vi "AccelerometerTest.vi"() -> ()   [LabVIEW 2016]
uses:
  Telemetry/TelemetryFields.ctl
  <vilib>/rvi/Emulation/niFpgaGetClockAttributes.vi
  <vilib>/rvi/Emulation/niFpgaSctlEmulationGetInTimedLoop.vi
  <vilib>/rvi/Emulation/niFpgaEmulationReportErrorSimple.vi
  <vilib>/rvi/Emulation/niFpgaEmulationIsFPGAContextNoSignature.vi
  <vilib>/rvi/errors/niFpgaSetErrorForExecOnDevCompSimple.vi
  <vilib>/rvi/eio/common/nirviEmuReportErrorAndStop.vi
  <vilib>/rvi/DataTransferAndStorage/Container/Common/niFpgaContainerGetUniqueNameForEmu.vi
  <vilib>/rvi/FIFO/Fifo_Resource/nirvififoEmulationSetSize.vi
  <vilib>/rvi/FIFO/Fifo_Resource/nirviFifoEmulationQueueMgr.vi
  <instcachedir>/0/nirviFifoEmulationQueueMgr_E5CAEC123FF24DC58D834DCA3CDAA9B5.lvgen/nirviFifoEmulationQueueMgr_E5CAEC123FF24DC58D834DCA3CDAA9B5_004.vi
  <vilib>/rvi/FIFO/Fifo_Resource/nirvififoEmulationDetermineInputValidOut.vi
  <vilib>/rvi/FIFO/Fifo_Resource/nirvififoEmulationCreateLock.vi
  <vilib>/rvi/Emulation/niFpgaProcessEmulError.vi
  <vilib>/rvi/FIFO/Fifo_Resource/nirvififoEmulationObtainLock.vi
  <vilib>/rvi/FIFO/Fifo_Resource/nirvififoEmulationReleaseLock.vi
  <vilib>/rvi/occurrence/nirviWaitOnOccurrenceBase.vi
  <vilib>/rvi/errors/nirviReportUnexpectedCaseInternalError.vi
  <vilib>/rvi/errors/nirviReportUnexpectedCaseInternalError (U32).vi
  <vilib>/Utility/error.llb/Clear Errors.vi
  <vilib>/rvi/Emulation/niFpgaCriticalErrorInLSC.vi
  <instcachedir>/0/nirviFifoEmulationQueueMgr_E5CAEC123FF24DC58D834DCA3CDAA9B5.lvgen/nirviFifoEmulationQueueMgr_E5CAEC123FF24DC58D834DCA3CDAA9B5_038.vi
  <instcachedir>/0/nirviFifoEmulationQueueMgr_E5CAEC123FF24DC58D834DCA3CDAA9B5.lvgen/nirviFifoEmulationQueueMgr_E5CAEC123FF24DC58D834DCA3CDAA9B5_039.vi
  <instcachedir>/0/nirviFifoEmulationQueueMgr_E5CAEC123FF24DC58D834DCA3CDAA9B5.lvgen/nirviFifoEmulationQueueMgr_E5CAEC123FF24DC58D834DCA3CDAA9B5_029.vi
  <instcachedir>/0/nirviFifoEmulationQueueMgr_E5CAEC123FF24DC58D834DCA3CDAA9B5.lvgen/nirviFifoEmulationQueueMgr_E5CAEC123FF24DC58D834DCA3CDAA9B5_028.vi
  <instcachedir>/0/nirviFifoEmulationQueueMgr_E5CAEC123FF24DC58D834DCA3CDAA9B5.lvgen/nirviFifoEmulationQueueMgr_E5CAEC123FF24DC58D834DCA3CDAA9B5_033.vi
  <instcachedir>/0/nirviFifoEmulationQueueMgr_E5CAEC123FF24DC58D834DCA3CDAA9B5.lvgen/nirviFifoEmulationQueueMgr_E5CAEC123FF24DC58D834DCA3CDAA9B5_035.vi
  <instcachedir>/0/nirviFifoEmulationQueueMgr_E5CAEC123FF24DC58D834DCA3CDAA9B5.lvgen/nirviFifoEmulationQueueMgr_E5CAEC123FF24DC58D834DCA3CDAA9B5_043.vi
  <instcachedir>/0/nirviFifoEmulationQueueMgr_E5CAEC123FF24DC58D834DCA3CDAA9B5.lvgen/nirviFifoEmulationQueueMgr_E5CAEC123FF24DC58D834DCA3CDAA9B5_041.vi
  <instcachedir>/0/nirviFifoEmulationQueueMgr_E5CAEC123FF24DC58D834DCA3CDAA9B5.lvgen/nirviFifoEmulationQueueMgr_E5CAEC123FF24DC58D834DCA3CDAA9B5_042.vi
  <instcachedir>/0/nirviFifoEmulationQueueMgr_E5CAEC123FF24DC58D834DCA3CDAA9B5.lvgen/nirviFifoEmulationQueueMgr_E5CAEC123FF24DC58D834DCA3CDAA9B5_040.vi
  <vilib>/rvi/DataTransferAndStorage/Container/XNode/niFpgaContainer.xnode
  <vilib>/rvi/FIFO/Fifo_Resource/nirvififoEmulationWrite.vi
  <vilib>/rvi/FIFO/Fifo_Resource/nirvififoEmulationRead.vi
panel:
  out "AngularAccelerationZ":sgl format="%#.6f"
  out "AngularAccelerationY":sgl format="%#.6f"
  out "AngularAccelerationX":sgl format="%#.6f"
  out "AccelerometerEng8":sgl format="%#.6f"
  out "AccelerometerEng7":sgl format="%#.6f"
  out "AccelerometerEng6":sgl format="%#.6f"
  out "AccelerometerEng5":sgl format="%#.6f"
  out "AccelerometerEng4":sgl format="%#.6f"
  out "AccelerometerEng3":sgl format="%#.6f"
  out "AccelerometerEng2":sgl format="%#.6f"
  out "AccelerometerEng1":sgl format="%#.6f"
  out "AccelerometerTimestamp":u64
  out "AccelerometerRaw1":sgl format="%#.6f"
  out "AccelerometerRaw2":sgl format="%#.6f"
  out "AccelerometerRaw3":sgl format="%#.6f"
  out "AccelerometerRaw4":sgl format="%#.6f"
  out "AccelerometerRaw5":sgl format="%#.6f"
  out "AccelerometerRaw6":sgl format="%#.6f"
  out "AccelerometerRaw7":sgl format="%#.6f"
  out "AccelerometerRaw8":sgl format="%#.6f"
  out "AccelerometerSampleCount":u64
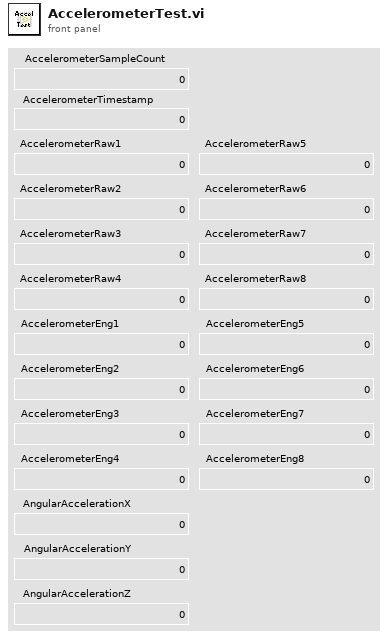
[diagram p1: front panel]
types:
  T1 = cluster{"Timestamp":u64, "TxBytes":u64, "RxBytes":u64, "TxFrames":u64, "RxFrames":u64, "BIT0":u8, "BIT1":u8, "BIT2":u8, "BIT3":u8, "BIT4":u8, "BIT5":u8}
  T2 = cluster{"Timestamp":u64, "TxBytes":u64, "RxBytes":u64, "TxFrames":u64, "RxFrames":u64, "GyroX":u32, "GyroY":u32, "GyroZ":u32, "Status":u8, "SequenceNumber":u8, "Temperature":i16}
  T3 = cluster{"Timestamp":u64, "TxBytes":u64, "RxBytes":u64, "TxFrames":u64, "RxFrames":u64, "BIT0":u8, "BIT1":u8, "BIT2":u8, "BIT3":u8, "BIT4":u8, "BIT5":u8, "BIT6":u8, "BIT7":u8}
  T4 = cluster{"Timestamp":u64, "TxBytes":u64, "RxBytes":u64, "TxFrames":u64, "RxFrames":u64, "ErrorCode":enum8{"None", "ResponseHeaderError", "ResponseCRCError", "ResponseTimeoutError", "ResponseChecksumError"}}
  T5 = cluster{"Timestamp":u64, "TxBytes":u64, "RxBytes":u64, "TxFrames":u64, "RxFrames":u64, "RawAngle":i32, "ZenithAngle":sgl}
  T6 = cluster{"Timestamp":u64, "TxBytes":u64, "RxBytes":u64, "TxFrames":u64, "RxFrames":u64, "ErrorCode":enum8{"None", "ResponseAddressError", "ResponseFunctionCodeError", "ResponseByteCountError", "ResponseCRCError", "ResponseUnknownError", "ResponseTimeoutError", "SensorReportsIllegalFunction", "SensorReportsIllegalDataAddress"}}
  T7 = cluster{"Timestamp":u64, "TxBytes":u64, "RxBytes":u64, "TxFrames":u64, "RxFrames":u64, "Sensor1Raw":i32, "Sensor2Raw":i32, "Sensor3Raw":i32, "Sensor4Raw":i32, "Sensor5Raw":i32, "Sensor6Raw":i32, "Sensor7Raw":i32, "Sensor8Raw":i32, "Sensor1Eng":sgl, "Sensor2Eng":sgl, "Sensor3Eng":sgl, "Sensor4Eng":sgl, "Sensor5Eng":sgl, "Sensor6Eng":sgl, "Sensor7Eng":sgl, "Sensor8Eng":sgl, "PositionX":sgl, "PositionY":sgl, "PositionZ":sgl, "RotationX":sgl, "RotationY":sgl, "RotationZ":sgl}
  T8 = cluster{"Timestamp":u64, "TxBytes":u64, "RxBytes":u64, "TxFrames":u64, "RxFrames":u64, "ErrorCode":enum16{"None", "ResponseUnknownError", "ResponseInvalidError", "ResponseTimeoutError", "SensorIndicatesInvalidCommandError", "SensorIndicatesCommunicationTimeoutError", "SensorIndicatesDataLengthError", "SensorIndicatesNumberOfParametersError", "SensorIndicatesParameterError", "SensorIndicatesCommunicationError", "SensorIndicatesIDNumberError", "SensorIndicatesExpansionLineError", "SensorIndicatesWriteControlError"}}
  T9 = typedef "TelemetryFields.ctl" = enum16{"None", "InclinometerTxBytes", "InclinometerRxBytes", "InclinometerTxFrames", "InclinometerRxFrames", "InclinometerErrorTimestamp", "InclinometerErrorCode", "InclinometerSampleTimestamp", "InclinometerRawAngle", "InclinometerZenithAngle", "DisplacementTxBytes", "DisplacementRxBytes", "DisplacementTxFrames", "DisplacementRxFrames", "DisplacementErrorTimestamp", "DisplacementErrorCode", "DisplacementSampleTimestamp", "DisplacementRaw1", "DisplacementRaw2", "DisplacementRaw3", "DisplacementRaw4", "DisplacementRaw5", "DisplacementRaw6", "DisplacementRaw7", "DisplacementRaw8", "DisplacementEng1", "DisplacementEng2", "DisplacementEng3", "DisplacementEng4", "DisplacementEng5", "DisplacementEng6", "DisplacementEng7", "DisplacementEng8", "DisplacementPositionX", "DisplacementPositionY", "DisplacementPositionZ", "DisplacementRotationX", "DisplacementRotationY", "DisplacementRotationZ", "AccelerometerSampleCount", "AccelerometerSampleTimestamp", "AccelerometerRaw1", "AccelerometerRaw2", "AccelerometerRaw3", "AccelerometerRaw4", "AccelerometerRaw5", "AccelerometerRaw6", "AccelerometerRaw7", "AccelerometerRaw8", "AccelerometerEng1", "AccelerometerEng2", "AccelerometerEng3", "AccelerometerEng4", "AccelerometerEng5", "AccelerometerEng6", "AccelerometerEng7", "AccelerometerEng8", "AngularAccelerationX", "AngularAccelerationY", "AngularAccelerationZ", "GyroTxBytes", "GyroRxBytes", "GyroTxFrames", "GyroRxFrames", "GyroErrorTimestamp", "GyroErrorCode", "GyroSampleTimestamp", "AngularVelocityX", "AngularVelocityY", "AngularVelocityZ", "GyroStatus", "GyroSequenceNumber", "GyroTemperature", "GyroBITTimestamp", "GyroBIT0", "GyroBIT1", "GyroBIT2", "GyroBIT3", "GyroBIT4", "GyroBIT5", "GyroBIT6", "GyroBIT7"}
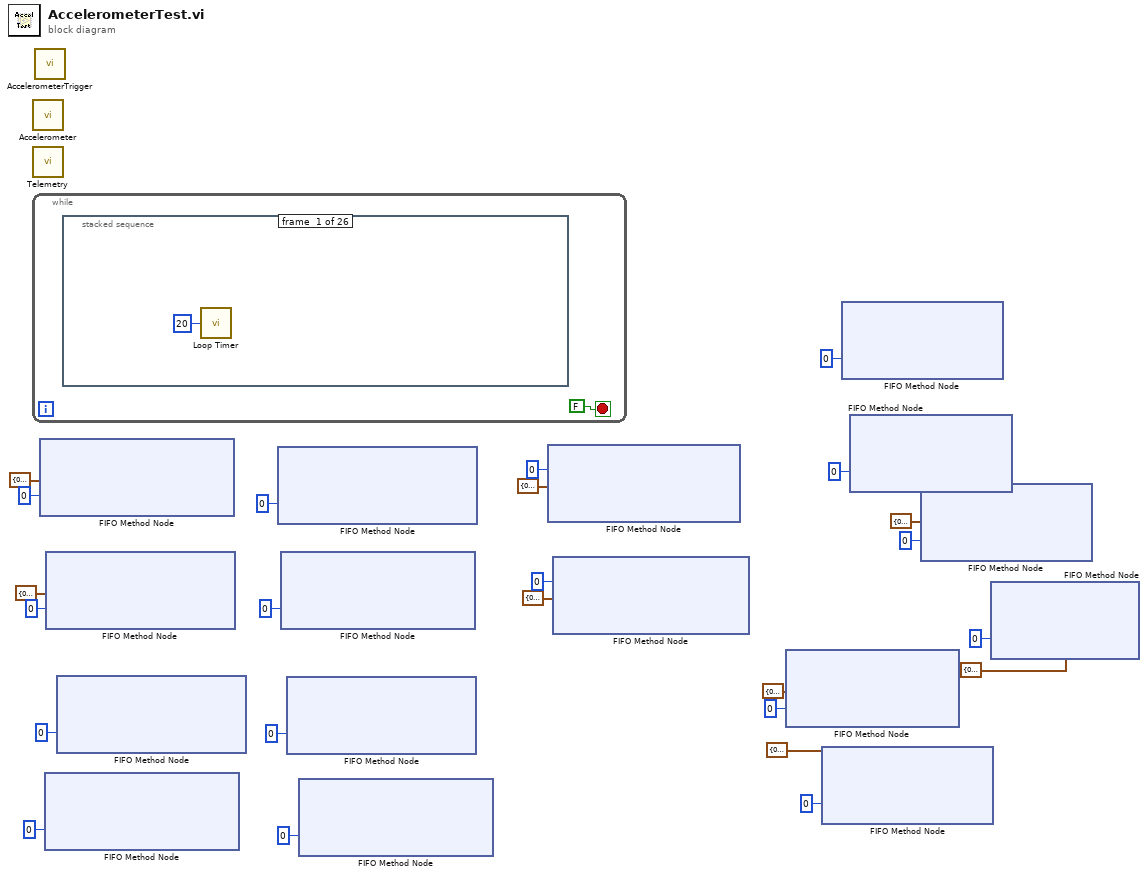
[diagram p0: block diagram]
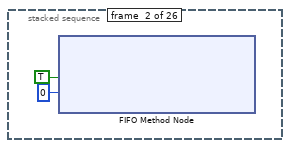
[diagram p2: hidden frame]
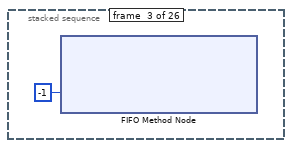
[diagram p3: hidden frame]
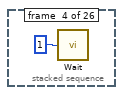
[diagram p4: hidden frame]
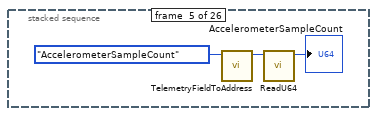
[diagram p5: hidden frame]
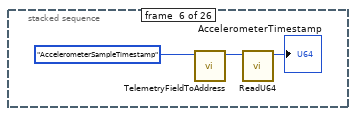
[diagram p6: hidden frame]
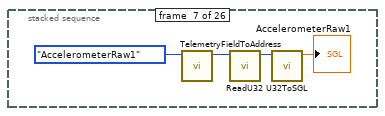
[diagram p7: hidden frame]
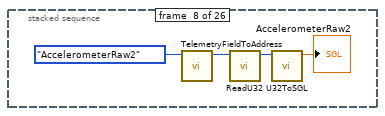
[diagram p8: hidden frame]
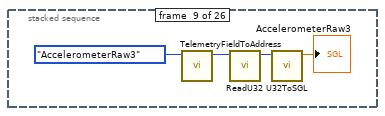
[diagram p9: hidden frame]
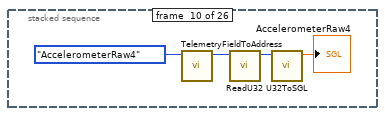
[diagram p10: hidden frame]
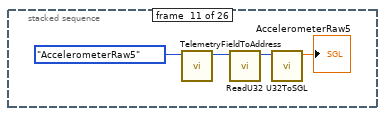
[diagram p11: hidden frame]
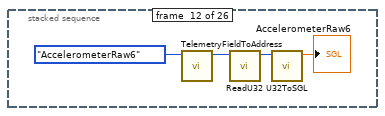
[diagram p12: hidden frame]
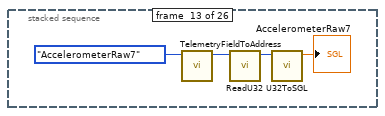
[diagram p13: hidden frame]
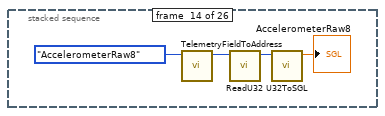
[diagram p14: hidden frame]
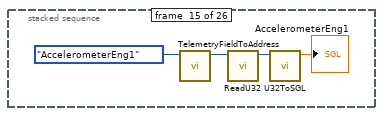
[diagram p15: hidden frame]
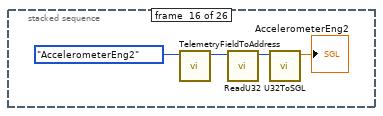
[diagram p16: hidden frame]
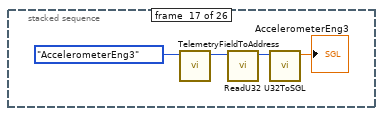
[diagram p17: hidden frame]
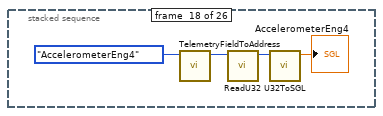
[diagram p18: hidden frame]
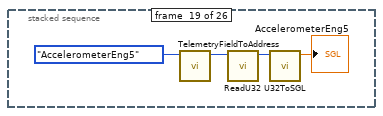
[diagram p19: hidden frame]
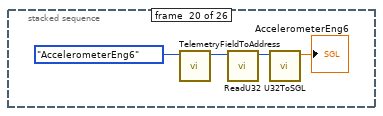
[diagram p20: hidden frame]
diagram:
  n1 = call "Accelerometer.vi"() -> ()  [unwired: 12 in]
  n2 = call "Telemetry.vi"() -> ()  [unwired: 12 in]
  n3 = while {
    stop <- FALSE stop-if-true
    n4 = stacked-sequence {
      frame #0 {
        n5 = call "Loop Timer"("Count(mSec)"=u8 20) -> ()  [unwired: 1 out]
      }
      frame #1 {
        n6 = xnode ("FIFO Method Node")("Element"=TRUE, "Timeout"=0) -> ()  [unwired: 1 in, 2 out]
      }
      frame #2 {
        n7 = xnode ("FIFO Method Node")("Timeout"=-1) -> ()  [unwired: 1 in, 3 out]
      }
      frame #3 {
        n8 = call "Wait"("Count(uSec)"=u8 1 ("Count(mSec)")) -> ()  [unwired: 1 out]
      }
      frame #4 {
        n9 = call "TelemetryFieldToAddress.vi"("TelemetryFields"=TelemetryFields."AccelerometerSampleCount") -> ("Address"=w32:u32)  [unwired: 10 in]
        n10 = call "ReadU64.vi"("Address"=w32) -> ("Data"=→"AccelerometerSampleCount":u64)  [unwired: 10 in]
      }
      frame #5 {
        n11 = call "TelemetryFieldToAddress.vi"("TelemetryFields"=TelemetryFields."AccelerometerSampleTimestamp") -> ("Address"=w36:u32)  [unwired: 10 in]
        n12 = call "ReadU64.vi"("Address"=w36) -> ("Data"=→"AccelerometerTimestamp":u64)  [unwired: 10 in]
      }
      frame #6 {
        n13 = call "TelemetryFieldToAddress.vi"("TelemetryFields"=TelemetryFields."AccelerometerRaw1") -> ("Address"=w40:u32)  [unwired: 10 in]
        n14 = call "ReadU32.vi"("Address"=w40) -> ("Data"=w39:u32)  [unwired: 10 in]
        n15 = call "U32ToSGL.vi"("U32"=w39) -> ("SGL"=→"AccelerometerRaw1":sgl)  [unwired: 10 in]
      }
      frame #7 {
        n16 = call "TelemetryFieldToAddress.vi"("TelemetryFields"=TelemetryFields."AccelerometerRaw2") -> ("Address"=w44:u32)  [unwired: 10 in]
        n17 = call "ReadU32.vi"("Address"=w44) -> ("Data"=w43:u32)  [unwired: 10 in]
        n18 = call "U32ToSGL.vi"("U32"=w43) -> ("SGL"=→"AccelerometerRaw2":sgl)  [unwired: 10 in]
      }
      frame #8 {
        n19 = call "TelemetryFieldToAddress.vi"("TelemetryFields"=TelemetryFields."AccelerometerRaw3") -> ("Address"=w48:u32)  [unwired: 10 in]
        n20 = call "ReadU32.vi"("Address"=w48) -> ("Data"=w47:u32)  [unwired: 10 in]
        n21 = call "U32ToSGL.vi"("U32"=w47) -> ("SGL"=→"AccelerometerRaw3":sgl)  [unwired: 10 in]
      }
      frame #9 {
        n22 = call "TelemetryFieldToAddress.vi"("TelemetryFields"=TelemetryFields."AccelerometerRaw4") -> ("Address"=w52:u32)  [unwired: 10 in]
        n23 = call "ReadU32.vi"("Address"=w52) -> ("Data"=w51:u32)  [unwired: 10 in]
        n24 = call "U32ToSGL.vi"("U32"=w51) -> ("SGL"=→"AccelerometerRaw4":sgl)  [unwired: 10 in]
      }
      frame #10 {
        n25 = call "TelemetryFieldToAddress.vi"("TelemetryFields"=TelemetryFields."AccelerometerRaw5") -> ("Address"=w56:u32)  [unwired: 10 in]
        n26 = call "ReadU32.vi"("Address"=w56) -> ("Data"=w55:u32)  [unwired: 10 in]
        n27 = call "U32ToSGL.vi"("U32"=w55) -> ("SGL"=→"AccelerometerRaw5":sgl)  [unwired: 10 in]
      }
      frame #11 {
        n28 = call "TelemetryFieldToAddress.vi"("TelemetryFields"=TelemetryFields."AccelerometerRaw6") -> ("Address"=w60:u32)  [unwired: 10 in]
        n29 = call "ReadU32.vi"("Address"=w60) -> ("Data"=w59:u32)  [unwired: 10 in]
        n30 = call "U32ToSGL.vi"("U32"=w59) -> ("SGL"=→"AccelerometerRaw6":sgl)  [unwired: 10 in]
      }
      frame #12 {
        n31 = call "TelemetryFieldToAddress.vi"("TelemetryFields"=TelemetryFields."AccelerometerRaw7") -> ("Address"=w64:u32)  [unwired: 10 in]
        n32 = call "ReadU32.vi"("Address"=w64) -> ("Data"=w63:u32)  [unwired: 10 in]
        n33 = call "U32ToSGL.vi"("U32"=w63) -> ("SGL"=→"AccelerometerRaw7":sgl)  [unwired: 10 in]
      }
      frame #13 {
        n34 = call "TelemetryFieldToAddress.vi"("TelemetryFields"=TelemetryFields."AccelerometerRaw8") -> ("Address"=w68:u32)  [unwired: 10 in]
        n35 = call "ReadU32.vi"("Address"=w68) -> ("Data"=w67:u32)  [unwired: 10 in]
        n36 = call "U32ToSGL.vi"("U32"=w67) -> ("SGL"=→"AccelerometerRaw8":sgl)  [unwired: 10 in]
      }
      frame #14 {
        n37 = call "TelemetryFieldToAddress.vi"("TelemetryFields"=TelemetryFields."AccelerometerEng1") -> ("Address"=w72:u32)  [unwired: 10 in]
        n38 = call "ReadU32.vi"("Address"=w72) -> ("Data"=w71:u32)  [unwired: 10 in]
        n39 = call "U32ToSGL.vi"("U32"=w71) -> ("SGL"=→"AccelerometerEng1":sgl)  [unwired: 10 in]
      }
      frame #15 {
        n40 = call "TelemetryFieldToAddress.vi"("TelemetryFields"=TelemetryFields."AccelerometerEng2") -> ("Address"=w76:u32)  [unwired: 10 in]
        n41 = call "ReadU32.vi"("Address"=w76) -> ("Data"=w75:u32)  [unwired: 10 in]
        n42 = call "U32ToSGL.vi"("U32"=w75) -> ("SGL"=→"AccelerometerEng2":sgl)  [unwired: 10 in]
      }
      frame #16 {
        n43 = call "TelemetryFieldToAddress.vi"("TelemetryFields"=TelemetryFields."AccelerometerEng3") -> ("Address"=w80:u32)  [unwired: 10 in]
        n44 = call "ReadU32.vi"("Address"=w80) -> ("Data"=w79:u32)  [unwired: 10 in]
        n45 = call "U32ToSGL.vi"("U32"=w79) -> ("SGL"=→"AccelerometerEng3":sgl)  [unwired: 10 in]
      }
      frame #17 {
        n46 = call "TelemetryFieldToAddress.vi"("TelemetryFields"=TelemetryFields."AccelerometerEng4") -> ("Address"=w84:u32)  [unwired: 10 in]
        n47 = call "ReadU32.vi"("Address"=w84) -> ("Data"=w83:u32)  [unwired: 10 in]
        n48 = call "U32ToSGL.vi"("U32"=w83) -> ("SGL"=→"AccelerometerEng4":sgl)  [unwired: 10 in]
      }
      frame #18 {
        n49 = call "TelemetryFieldToAddress.vi"("TelemetryFields"=TelemetryFields."AccelerometerEng5") -> ("Address"=w88:u32)  [unwired: 10 in]
        n50 = call "ReadU32.vi"("Address"=w88) -> ("Data"=w87:u32)  [unwired: 10 in]
        n51 = call "U32ToSGL.vi"("U32"=w87) -> ("SGL"=→"AccelerometerEng5":sgl)  [unwired: 10 in]
      }
      frame #19 {
        n52 = call "TelemetryFieldToAddress.vi"("TelemetryFields"=TelemetryFields."AccelerometerEng6") -> ("Address"=w92:u32)  [unwired: 10 in]
        n53 = call "ReadU32.vi"("Address"=w92) -> ("Data"=w91:u32)  [unwired: 10 in]
        n54 = call "U32ToSGL.vi"("U32"=w91) -> ("SGL"=→"AccelerometerEng6":sgl)  [unwired: 10 in]
      }
      frame #20 {
        n55 = call "TelemetryFieldToAddress.vi"("TelemetryFields"=TelemetryFields."AccelerometerEng7") -> ("Address"=w96:u32)  [unwired: 10 in]
        n56 = call "ReadU32.vi"("Address"=w96) -> ("Data"=w95:u32)  [unwired: 10 in]
        n57 = call "U32ToSGL.vi"("U32"=w95) -> ("SGL"=→"AccelerometerEng7":sgl)  [unwired: 10 in]
      }
      frame #21 {
        n58 = call "TelemetryFieldToAddress.vi"("TelemetryFields"=TelemetryFields."AccelerometerEng8") -> ("Address"=w100:u32)  [unwired: 10 in]
        n59 = call "ReadU32.vi"("Address"=w100) -> ("Data"=w99:u32)  [unwired: 10 in]
        n60 = call "U32ToSGL.vi"("U32"=w99) -> ("SGL"=→"AccelerometerEng8":sgl)  [unwired: 10 in]
      }
      frame #22 {
        n61 = call "TelemetryFieldToAddress.vi"("TelemetryFields"=TelemetryFields."AngularAccelerationX") -> ("Address"=w104:u32)  [unwired: 10 in]
        n62 = call "ReadU32.vi"("Address"=w104) -> ("Data"=w103:u32)  [unwired: 10 in]
        n63 = call "U32ToSGL.vi"("U32"=w103) -> ("SGL"=→"AngularAccelerationX":sgl)  [unwired: 10 in]
      }
      frame #23 {
        n64 = call "TelemetryFieldToAddress.vi"("TelemetryFields"=TelemetryFields."AngularAccelerationY") -> ("Address"=w108:u32)  [unwired: 10 in]
        n65 = call "ReadU32.vi"("Address"=w108) -> ("Data"=w107:u32)  [unwired: 10 in]
        n66 = call "U32ToSGL.vi"("U32"=w107) -> ("SGL"=→"AngularAccelerationY":sgl)  [unwired: 10 in]
      }
      frame #24 {
        n67 = call "TelemetryFieldToAddress.vi"("TelemetryFields"=TelemetryFields."AngularAccelerationZ") -> ("Address"=w112:u32)  [unwired: 10 in]
        n68 = call "ReadU32.vi"("Address"=w112) -> ("Data"=w111:u32)  [unwired: 10 in]
        n69 = call "U32ToSGL.vi"("U32"=w111) -> ("SGL"=→"AngularAccelerationZ":sgl)  [unwired: 10 in]
      }
      frame #25 {
        n70 = xnode ("FIFO Method Node")("Element"=TRUE, "Timeout"=0) -> ()  [unwired: 1 in, 2 out]
      }
    }
  }
  n71 = call "AccelerometerTrigger.vi"() -> ()  [unwired: 12 in]
  n72 = xnode ("FIFO Method Node")("Element"=T8 {"Timestamp"=0, "TxBytes"=0, "RxBytes"=0, "TxFrames"=0, "RxFrames"=0, "ErrorCode"=enum."None"}, "Timeout"=0) -> ()  [unwired: 1 in, 2 out]
  n73 = xnode ("FIFO Method Node")("Timeout"=0) -> ()  [unwired: 1 in, 3 out]
  n74 = xnode ("FIFO Method Node")("Element"=T6 {"Timestamp"=0, "TxBytes"=0, "RxBytes"=0, "TxFrames"=0, "RxFrames"=0, "ErrorCode"=enum."None"}, "Timeout"=0) -> ()  [unwired: 1 in, 2 out]
  n75 = xnode ("FIFO Method Node")("Timeout"=0) -> ()  [unwired: 1 in, 3 out]
  n76 = xnode ("FIFO Method Node")("Timeout"=0) -> ()  [unwired: 1 in, 3 out]
  n77 = xnode ("FIFO Method Node")("Timeout"=0) -> ()  [unwired: 1 in, 3 out]
  n78 = xnode ("FIFO Method Node")("Timeout"=0) -> ()  [unwired: 1 in, 3 out]
  n79 = xnode ("FIFO Method Node")("Timeout"=0) -> ()  [unwired: 1 in, 3 out]
  n80 = xnode ("FIFO Method Node")("Element"=T7 {"Timestamp"=0, "TxBytes"=0, "RxBytes"=0, "TxFrames"=0, "RxFrames"=0, "Sensor1Raw"=0, "Sensor2Raw"=0, "Sensor3Raw"=0, "Sensor4Raw"=0, "Sensor5Raw"=0, "Sensor6Raw"=0, "Sensor7Raw"=0, "Sensor8Raw"=0, "Sensor1Eng"=0.0, "Sensor2Eng"=0.0, "Sensor3Eng"=0.0, "Sensor4Eng"=0.0, "Sensor5Eng"=0.0, "Sensor6Eng"=0.0, "Sensor7Eng"=0.0, "Sensor8Eng"=0.0, "PositionX"=0.0, "PositionY"=0.0, "PositionZ"=0.0, "RotationX"=0.0, "RotationY"=0.0, "RotationZ"=0.0}, "Timeout"=0) -> ()  [unwired: 1 in, 2 out]
  n81 = xnode ("FIFO Method Node")("Element"=T5 {"Timestamp"=0, "TxBytes"=0, "RxBytes"=0, "TxFrames"=0, "RxFrames"=0, "RawAngle"=0, "ZenithAngle"=0.0}, "Timeout"=0) -> ()  [unwired: 1 in, 2 out]
  n82 = xnode ("FIFO Method Node")("Element"=T4 {"Timestamp"=0, "TxBytes"=0, "RxBytes"=0, "TxFrames"=0, "RxFrames"=0, "ErrorCode"=enum."None"}, "Timeout"=0) -> ()  [unwired: 1 in, 2 out]
  n83 = xnode ("FIFO Method Node")("Element"=T1 {"Timestamp"=0, "TxBytes"=0, "RxBytes"=0, "TxFrames"=0, "RxFrames"=0, "BIT0"=0, "BIT1"=0, "BIT2"=0, "BIT3"=0, "BIT4"=0, "BIT5"=0}, "Timeout"=0) -> ()  [unwired: 1 in, 2 out]
  n84 = xnode ("FIFO Method Node")("Timeout"=0) -> ()  [unwired: 1 in, 3 out]
  n85 = xnode ("FIFO Method Node")("Timeout"=0) -> ()  [unwired: 1 in, 3 out]
  n86 = xnode ("FIFO Method Node")("Element"=T3 {"Timestamp"=0, "TxBytes"=0, "RxBytes"=0, "TxFrames"=0, "RxFrames"=0, "BIT0"=0, "BIT1"=0, "BIT2"=0, "BIT3"=0, "BIT4"=0, "BIT5"=0, "BIT6"=0, "BIT7"=0}, "Timeout"=0) -> ()  [unwired: 1 in, 2 out]
  n87 = xnode ("FIFO Method Node")("Element"=T2 {"Timestamp"=0, "TxBytes"=0, "RxBytes"=0, "TxFrames"=0, "RxFrames"=0, "GyroX"=0, "GyroY"=0, "GyroZ"=0, "Status"=0, "SequenceNumber"=0, "Temperature"=0}, "Timeout"=0) -> ()  [unwired: 1 in, 2 out]
